vi "Create.vi"(10 "Channel":refnum<class "StringChannel.lvclass">) -> (3 "ChannelValue out":refnum<class "StringChannelValue.lvclass">)   [LabVIEW 2020, in "Vecto.lvlib" / "StringChannelValue.lvclass"]
uses:
  StringChannelValue.lvclass
  StringChannelValue.lvclass/StringChannelValue.ctl
  StringChannel/StringChannel.lvclass
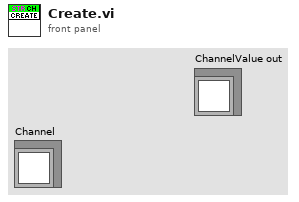
[diagram p1: front panel]
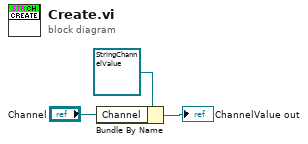
[diagram p0: block diagram]
diagram:
  n1 = Bundle By Name(cluster=refnum<class "StringChannelValue.lvclass"> refnum ("ChannelValue in"), "Channel"="Channel") -> (→"ChannelValue out":refnum<class "StringChannelValue.lvclass">)
